vi "Write Limiter Msg.vi"(8 "error in (no error)":errorcluster, 10 "Limiter":dbl, 11 "Helm Limiter Msg in":refnum<class "Helm Limiter Msg.lvclass">) -> (0 "error out":errorcluster, 3 "Helm Limiter Msg out":refnum<class "Helm Limiter Msg.lvclass">)   [LabVIEW 2015, in "RDS Child Messages.lvlib" / "Helm Limiter Msg.lvclass"]
uses:
  Helm Limiter Msg.lvclass
  Helm Limiter Msg.lvclass/Helm Limiter Msg.ctl
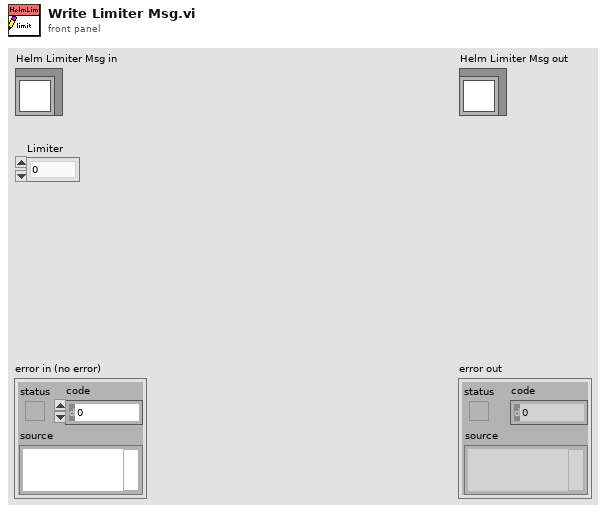
[diagram p1: front panel]
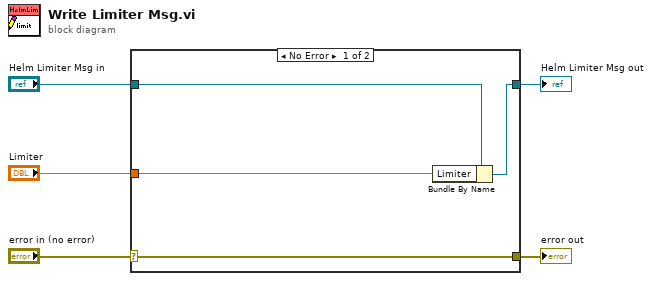
[diagram p0: block diagram]
diagram:
  n1 = case shown="No Error" "error in (no error)" {
    selector: "error in (no error)" -> [w9 w10]
    tunnel: [w9 w10] -> w4
    tunnel: [w7 w11] -> w2
    tunnel: "Helm Limiter Msg in" -> [w8 w11]
    tunnel: "Limiter" -> [w6 _]
    frame No Error {
      n2 = Bundle By Name(cluster=w8, "Limiter"=w6) -> (w7:refnum<class "Helm Limiter Msg.lvclass">)
    }
    frame Error {
    }
  }
  "error out" <- w4
  "Helm Limiter Msg out" <- w2
